vi "XiXi-1(Divide DBL[]).vi"(10 "X[-1]":dbl[](array[numeric]), 11 "Xi":dbl[][](array[numeric])) -> (2 "小数":dbl[][](array[numeric]), 3 "Yi":dbl[][](array[numeric]))   [LabVIEW 2012]
doc: "Calculate sums of consecutive array elements. 0th element of output is equal to x(0)+ x(-1), where x(-1) is an optional scalar input that defaults to zero."
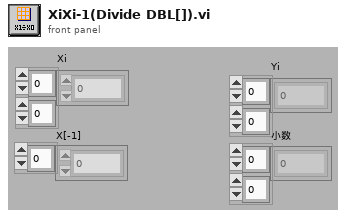
[diagram p1: front panel]
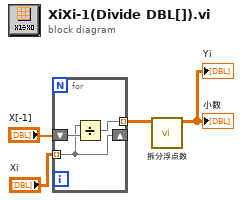
[diagram p0: block diagram]
diagram:
  n1 = for {
    shift-right: [w6] -> _
    shift-left: "X[-1]" -> [w7]
    tunnel: "Xi" -> [w6] mode=indexing
    tunnel: [w5] -> w1 mode=indexing
    n2 = Divide(x=w6, y=w7) -> (x/y=w5:dbl[])
  }
  n3 = call-poly "拆分浮点数.vi"("输入"=w1) -> ("整数部分"=→"Yi" →"小数":dbl[][])  [unwired: 9 in, 1 out]
